vi "VALEW_ATC_Wait for bath temp update.vi"(7 "ATC Data":T1) -> (4 "Bath temp updated after segment fill?":bool, 6 "Report Text":string, 8 "Bath temp after seg gals":dbl, 10 "Calc bath temp after seg gals":dbl)   [LabVIEW 2016, in "Centauro.lvlib"]
uses:
  Projects/Centauro.lvlib
  typedefs/VALEW_ATC_Data.ctl
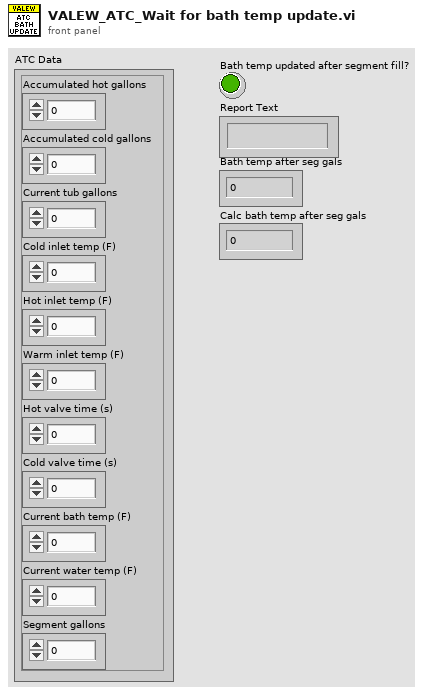
[diagram p1: front panel]
types:
  T1 = typedef "Centauro.lvlib/VALEW_ATC_Data.ctl" = cluster{"Accumulated hot gallons":dbl, "Accumulated cold gallons":dbl, "Current tub gallons":dbl, "Cold inlet temp (F)":dbl, "Hot inlet temp (F)":dbl, "Warm inlet temp (F)":dbl, "Hot valve time (s)":u16, "Cold valve time (s)":u16, "Current bath temp (F)":dbl, "Current water temp (F)":dbl, "Segment gallons":dbl}
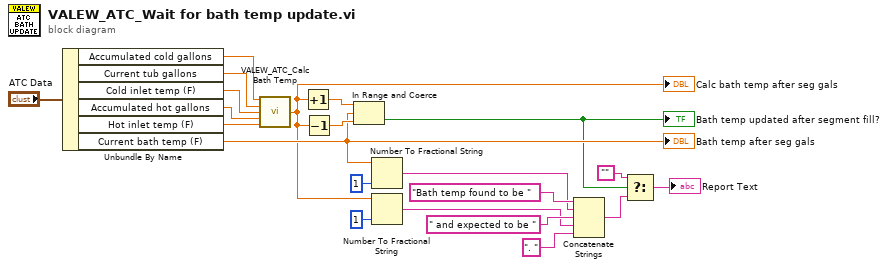
[diagram p0: block diagram]
diagram:
  n1 = Unbundle By Name("ATC Data") -> ("Accumulated cold gallons"=w17:dbl, "Current tub gallons"=w18:dbl, "Cold inlet temp (F)"=w19:dbl, "Accumulated hot gallons"=w20:dbl, "Hot inlet temp (F)"=w21:dbl, "Current bath temp (F)"=w8:dbl)
  "Bath temp after seg gals" <- w8
  n2 = call "VALEW_ATC_Calc Bath Temp.vi"("V(bath cold)"=w17, "V(bath)"=w18, "T(cold inlet)"=w19, "V(bath hot)"=w20, "T(hot inlet)"=w21) -> ("T(bath)"=w7:dbl)  [unwired: 10 in]
  "Calc bath temp after seg gals" <- w7
  n3 = Increment(x=w7) -> (x+1=w15:dbl)
  n4 = Decrement(x=w7) -> (x-1=w16:dbl)
  n5 = In Range and Coerce(upper limit=w15, x=w8, lower limit=w16) -> (In Range?=w3:bool)  [unwired: 1 out]
  "Bath temp updated after segment fill?" <- w3
  n6 = Number To Fractional String(number=w8, precision (6)=i16 1) -> (F-format string=w5:string)  [unwired: 2 in]
  n7 = Number To Fractional String(number=w7, precision (6)=i16 1) -> (F-format string=w4:string)  [unwired: 2 in]
  n8 = Concatenate Strings("Bath temp found to be ", w5, " and expected to be ", w4, ". " ("string")) -> (w9:string)
  n9 = Select(t="", s=w3, f=w9) -> (s? t:f=→"Report Text":string)
